vi "Add Rows.vi"(8 "error in (no error)":errorcluster, 10 "Cells":T2(array[cluster]), 11 "DataGridView in":refnum<class "DataGridView.lvclass">) -> (0 "error out":errorcluster, 3 "DataGridView out":refnum<class "DataGridView.lvclass">)   [LabVIEW 2013, in "DataGrid.lvlib" / "DataGridView.lvclass"]
doc: "This method allows you to add any rows of any time, regardless of the data column setup."
uses:
  DataGridView.lvclass
  GridColumn/ColumnType.ctl
  DataGridView.lvclass/DataGridView.ctl
  System.Windows.Forms
  DataTable/DataTable.lvclass
  GridColumn/GridColumn.lvclass
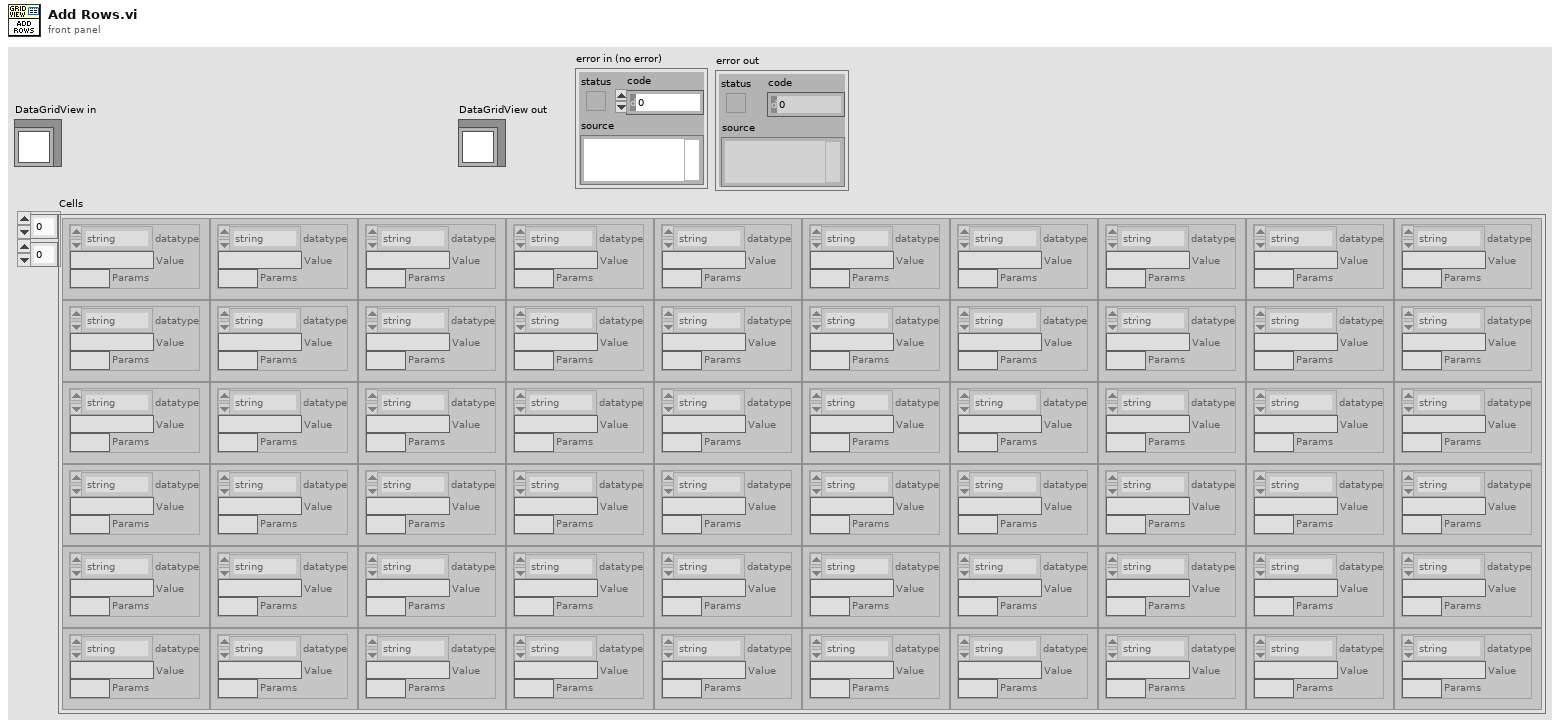
[diagram p1: front panel]
types:
  T1 = typedef "DataGrid.lvlib/GridColumn.lvclass/ColumnType.ctl" = enum16{"string", "image", "check", "numeric", "timestamp", "button", "combo", "link"}
  T2 = cluster{"datatype":T1, "Value":string, "Params":string}[][]
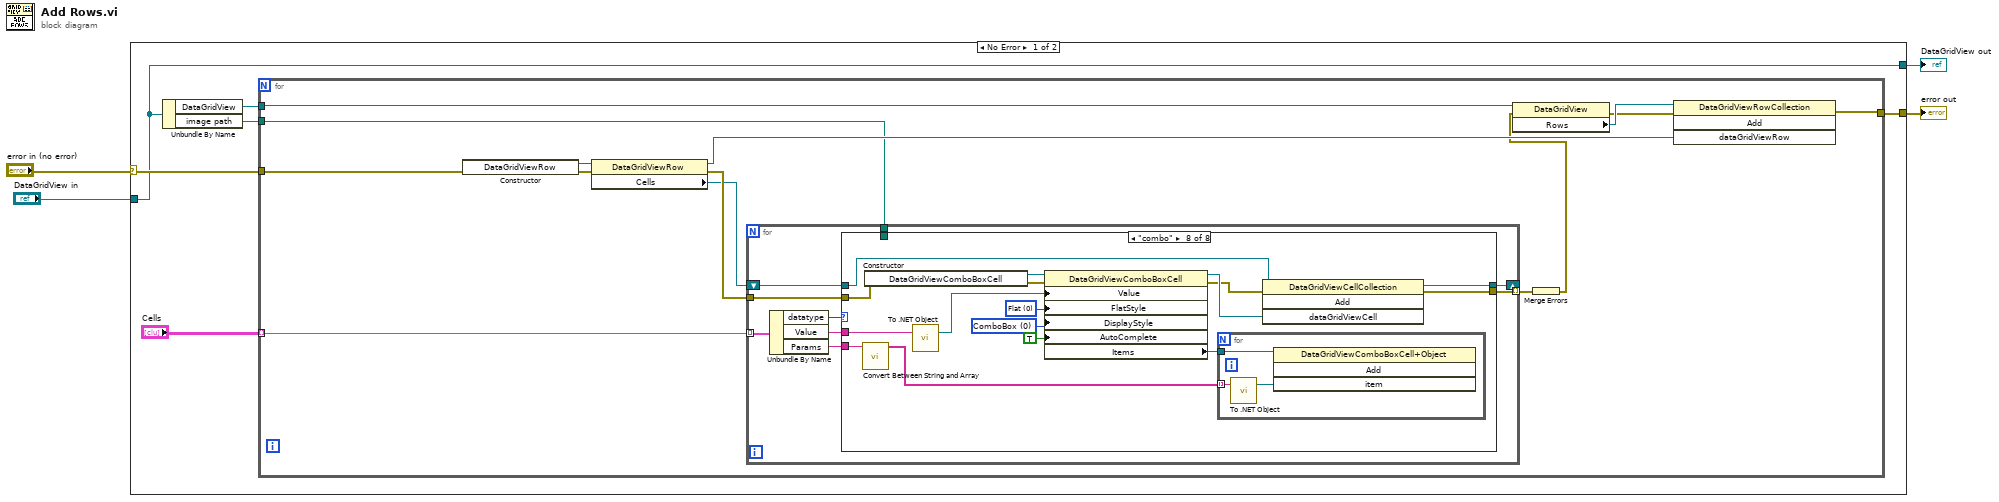
[diagram p0: block diagram]
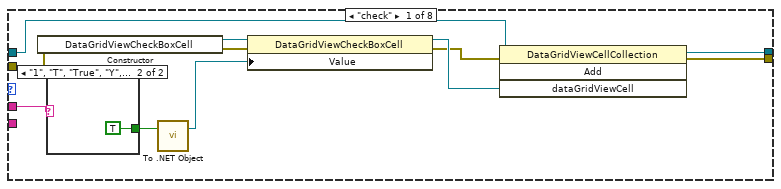
[diagram p2: hidden frame]
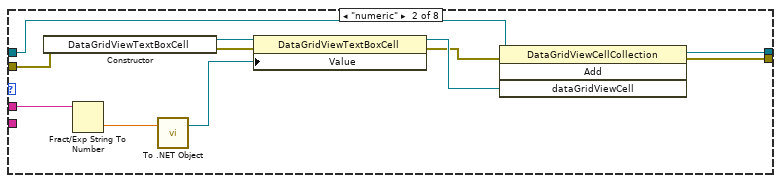
[diagram p4: hidden frame]
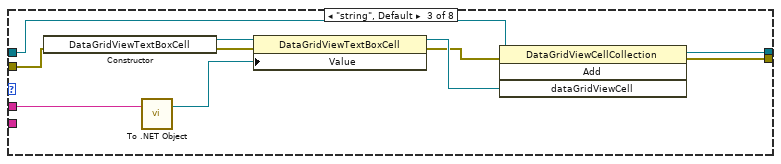
[diagram p5: hidden frame]
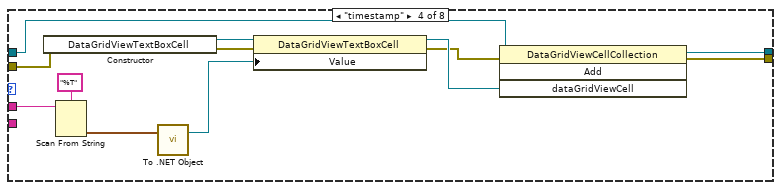
[diagram p6: hidden frame]
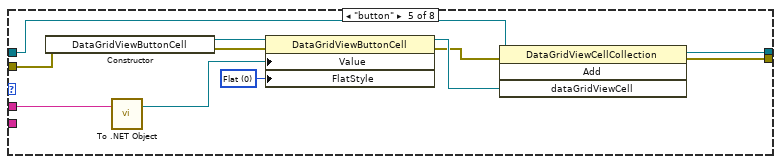
[diagram p7: hidden frame]
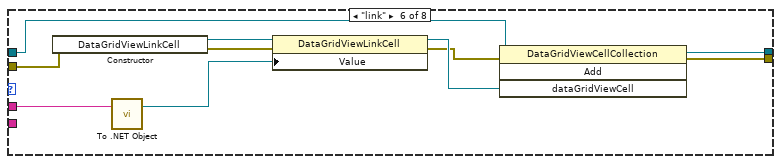
[diagram p8: hidden frame]
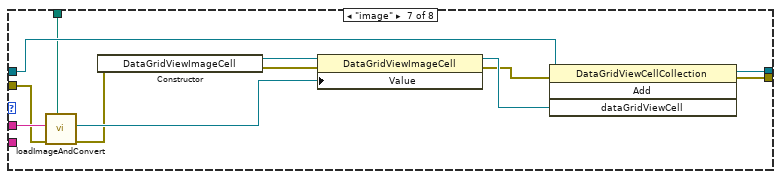
[diagram p9: hidden frame]
diagram:
  n1 = case shown="No Error" "error in (no error)" {
    selector: "error in (no error)" -> [w8 w132]
    tunnel: [w10 w132] -> w3
    tunnel: [w6 w131] -> w1
    tunnel: "DataGridView in" -> [w6 w131]
    frame No Error {
      n2 = Unbundle By Name(w6) -> ("DataGridView"=w9:refnum<k24>, "image path"=w5:path)
      n3 = for {
        tunnel: [w13] -> w10
        tunnel: w9 -> [w11]
        tunnel: w8 -> [w12]
        tunnel: "Cells" -> [w18] mode=indexing
        tunnel: w5 -> [w17]
        n4 = constructor class="DataGridViewRow"(error in=w12) -> (reference out=w22:refnum<k24>, error out=w23:errorcluster)  [unwired: 2 in, 1 out]
        n5 = property class="DataGridViewRow"(reference=w22, error in=w23) -> (reference out=w21:refnum<k24>, error out=w20:errorcluster, "Cells"=w19:refnum<k24>)
        n6 = for {
          tunnel: w18 -> [w33] mode=indexing
          shift-right: [w29] -> _
          shift-left: w19 -> [w28]
          tunnel: w20 -> [w27]
          tunnel: [w26] -> w24 mode=indexing
          tunnel: w17 -> [w25]
          n7 = Unbundle By Name(w33) -> ("datatype"=w32:T1, "Value"=w31:string, "Params"=w30:string)
          n8 = case shown="\"combo\"" w32 {
            tunnel: w31 -> [w43 w50 w60 w71 w82 w93 w106 w114]
            tunnel: w30 -> [_ _ _ _ _ _ _ w121]
            tunnel: [w40 w54 w64 w76 w87 w97 w109 w125] -> w29
            tunnel: w28 -> [w38 w52 w62 w74 w85 w95 w107 w123]
            tunnel: w27 -> [w36 w46 w59 w69 w79 w92 w102 w116]
            tunnel: [w34 w48 w57 w68 w80 w90 w104 w118] -> w26
            tunnel: w25 -> [_ _ _ _ _ _ w100 _]
            frame "check" {
              n9 = constructor class="DataGridViewCheckBoxCell"(error in=w36) -> (reference out=w41:refnum<k24>, error out=w42:errorcluster)  [unwired: 2 in, 1 out]
              n10 = case shown="\"1\", \"T\", \"True\", \"Y\", \"Yes\"" w43 {
                tunnel: [_ TRUE] -> w44
                frame Default {
                }
                frame "1", "T", "True", "Y", "Yes" {
                }
              }
              n11 = call <vilib>:"To .NET Object.vi"("anything"=w44) -> (".NET object"=w37:refnum<k24>)  [unwired: 1 in, 1 out]
              n12 = property class="DataGridViewCheckBoxCell"(reference=w41, error in=w42, "Value"=w37) -> (reference out=w39:refnum<k24>, error out=w35:errorcluster)
              n13 = invoke class="DataGridViewCellCollection" method="Add"(reference=w38, error in=w35, "dataGridViewCell"=w39) -> (reference out=w40:refnum<k24>, error out=w34:errorcluster)  [unwired: 1 in, 2 out]
            }
            frame "numeric" {
              n14 = constructor class="DataGridViewTextBoxCell"(error in=w46) -> (reference out=w55:refnum<k24>, error out=w56:errorcluster)  [unwired: 2 in, 1 out]
              n15 = Fract/Exp String To Number(string=w50) -> (number=w49:dbl)  [unwired: 3 in, 1 out]
              n16 = call <vilib>:"To .NET Object.vi"("anything"=w49) -> (".NET object"=w51:refnum<k24>)  [unwired: 1 in, 1 out]
              n17 = property class="DataGridViewTextBoxCell"(reference=w55, error in=w56, "Value"=w51) -> (reference out=w53:refnum<k24>, error out=w47:errorcluster)
              n18 = invoke class="DataGridViewCellCollection" method="Add"(reference=w52, error in=w47, "dataGridViewCell"=w53) -> (reference out=w54:refnum<k24>, error out=w48:errorcluster)  [unwired: 1 in, 2 out]
            }
            frame "string", Default {
              n19 = constructor class="DataGridViewTextBoxCell"(error in=w59) -> (reference out=w65:refnum<k24>, error out=w66:errorcluster)  [unwired: 2 in, 1 out]
              n20 = call <vilib>:"To .NET Object.vi"("anything"=w60) -> (".NET object"=w61:refnum<k24>)  [unwired: 1 in, 1 out]
              n21 = property class="DataGridViewTextBoxCell"(reference=w65, error in=w66, "Value"=w61) -> (reference out=w63:refnum<k24>, error out=w58:errorcluster)
              n22 = invoke class="DataGridViewCellCollection" method="Add"(reference=w62, error in=w58, "dataGridViewCell"=w63) -> (reference out=w64:refnum<k24>, error out=w57:errorcluster)  [unwired: 1 in, 2 out]
            }
            frame "timestamp" {
              n23 = constructor class="DataGridViewTextBoxCell"(error in=w69) -> (reference out=w77:refnum<k24>, error out=w78:errorcluster)  [unwired: 2 in, 1 out]
              n24 = Scan From String(format string="%T", input string=w71) -> (output 1=w70:timestamp)  [unwired: 3 in, 3 out]
              n25 = call <vilib>:"To .NET Object.vi"("anything"=w70) -> (".NET object"=w73:refnum<k24>)  [unwired: 1 in, 1 out]
              n26 = property class="DataGridViewTextBoxCell"(reference=w77, error in=w78, "Value"=w73) -> (reference out=w75:refnum<k24>, error out=w67:errorcluster)
              n27 = invoke class="DataGridViewCellCollection" method="Add"(reference=w74, error in=w67, "dataGridViewCell"=w75) -> (reference out=w76:refnum<k24>, error out=w68:errorcluster)  [unwired: 1 in, 2 out]
            }
            frame "button" {
              w83 = 0 items=["Flat", "Popup", "Standard", "System"] ("FlatStyle")
              n28 = constructor class="DataGridViewButtonCell"(error in=w79) -> (reference out=w88:refnum<k24>, error out=w89:errorcluster)  [unwired: 2 in, 1 out]
              n29 = call <vilib>:"To .NET Object.vi"("anything"=w82) -> (".NET object"=w84:refnum<k24>)  [unwired: 1 in, 1 out]
              n30 = property class="DataGridViewButtonCell"(reference=w88, error in=w89, "Value"=w84, "FlatStyle"=w83) -> (reference out=w86:refnum<k24>, error out=w81:errorcluster)
              n31 = invoke class="DataGridViewCellCollection" method="Add"(reference=w85, error in=w81, "dataGridViewCell"=w86) -> (reference out=w87:refnum<k24>, error out=w80:errorcluster)  [unwired: 1 in, 2 out]
            }
            frame "link" {
              n32 = constructor class="DataGridViewLinkCell"(error in=w92) -> (reference out=w98:refnum<k24>, error out=w99:errorcluster)  [unwired: 2 in, 1 out]
              n33 = call <vilib>:"To .NET Object.vi"("anything"=w93) -> (".NET object"=w94:refnum<k24>)  [unwired: 1 in, 1 out]
              n34 = property class="DataGridViewLinkCell"(reference=w98, error in=w99, "Value"=w94) -> (reference out=w96:refnum<k24>, error out=w91:errorcluster)
              n35 = invoke class="DataGridViewCellCollection" method="Add"(reference=w95, error in=w91, "dataGridViewCell"=w96) -> (reference out=w97:refnum<k24>, error out=w90:errorcluster)  [unwired: 1 in, 2 out]
            }
            frame "image" {
              n36 = call "loadImageAndConvert.vi"("image path"=w100, "error in (no error)"=w102, "name or relative path"=w106) -> ("error out"=w101:errorcluster, ".NET object"=w105:refnum<k24>)  [unwired: 7 in]
              n37 = constructor class="DataGridViewImageCell"(error in=w101) -> (reference out=w110:refnum<k24>, error out=w111:errorcluster)  [unwired: 2 in, 1 out]
              n38 = property class="DataGridViewImageCell"(reference=w110, error in=w111, "Value"=w105) -> (reference out=w108:refnum<k24>, error out=w103:errorcluster)
              n39 = invoke class="DataGridViewCellCollection" method="Add"(reference=w107, error in=w103, "dataGridViewCell"=w108) -> (reference out=w109:refnum<k24>, error out=w104:errorcluster)  [unwired: 1 in, 2 out]
            }
            frame "combo" {
              w119 = 0 items=["ComboBox", "DropDownButton", "Nothing"] ("DisplayStyle")
              w120 = 0 items=["Flat", "Popup", "Standard", "System"] ("FlatStyle")
              n40 = call "Convert Between String and Array.vi"("String"=w121) -> ("String Array"=w113:string[])  [unwired: 9 in, 1 out]
              n41 = constructor class="DataGridViewComboBoxCell"(error in=w116) -> (reference out=w126:refnum<k24>, error out=w127:errorcluster)  [unwired: 2 in, 1 out]
              n42 = call <vilib>:"To .NET Object.vi"("anything"=w114) -> (".NET object"=w122:refnum<k24>)  [unwired: 1 in, 1 out]
              n43 = property class="DataGridViewComboBoxCell"(reference=w126, error in=w127, "Value"=w122, "FlatStyle"=w120, "DisplayStyle"=w119, "AutoComplete"=TRUE) -> (reference out=w124:refnum<k24>, error out=w117:errorcluster, "Items"=w112:refnum<k24>)
              n44 = for {
                tunnel: w112 -> [w130]
                tunnel: w113 -> [w128] mode=indexing
                n45 = call <vilib>:"To .NET Object.vi"("anything"=w128) -> (".NET object"=w129:refnum<k24>)  [unwired: 1 in, 1 out]
                n46 = invoke class="DataGridViewComboBoxCell+Object" method="Add"(reference=w130, "item"=w129) -> ()  [unwired: 2 in, 4 out]
              }
              n47 = invoke class="DataGridViewCellCollection" method="Add"(reference=w123, error in=w117, "dataGridViewCell"=w124) -> (reference out=w125:refnum<k24>, error out=w118:errorcluster)  [unwired: 1 in, 2 out]
            }
          }
        }
        n48 = Merge Errors(w24) -> (w15:errorcluster)
        n49 = property class="DataGridView"(reference=w11, error in=w15) -> (error out=w14:errorcluster, "Rows"=w16:refnum<k24>)  [unwired: 1 out]
        n50 = invoke class="DataGridViewRowCollection" method="Add"(reference=w16, error in=w14, "dataGridViewRow"=w21) -> (error out=w13:errorcluster)  [unwired: 1 in, 3 out]
      }
    }
    frame Error {
    }
  }
  "error out" <- w3
  "DataGridView out" <- w1
